vi "Enable.vi"(0 "reference in":refnum<class "Battery.lvclass">, 2 "Enable":bool, 5 "Error In":errorcluster) -> (14 "reference out":refnum<class "Battery.lvclass">, 19 "Error Out":errorcluster)   [LabVIEW 2023, in "Battery.lvclass"]
uses:
  Battery.lvclass
  Battery.lvclass/Battery.ctl
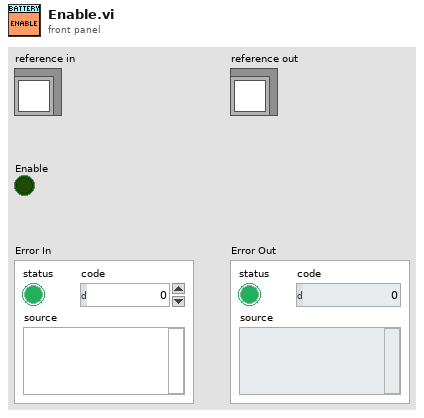
[diagram p1: front panel]
types:
  T1 = typedef "Battery.lvclass/ObjectAttributes.ctl" = cluster{"Python module":path, "Python Session":refnum<k35>, "PybammWrapper":refnum<k38>, "model loaded":bool, "simulation loaded":bool, "simulation enabled":bool, "SOC OCV Curve":dbl[][], "Open Circuit Voltage (V)":dbl, "State of Charge (%)":dbl, "HPS17K Refs":refnum<class "HPS-17000.lvclass">[], "# Cells in Series":u16, "# Cells in Parallel":u16, "Model Parameters":T2, "Simulation Parameters":T3}
  T2 = typedef "Battery.lvclass/Model Parameters.ctl" = cluster{"chemistry":string, "model_type":string}
  T3 = typedef "Battery.lvclass/Simulation Parameters.ctl" = cluster{"num_rc_pairs":i32, "R0":dbl, "R1":dbl, "C1":dbl, "R2":dbl, "C2":dbl, " nominal_capacity_Ah":dbl, "upper_voltage_cutoff":dbl, "lower_voltage_cutoff":dbl}
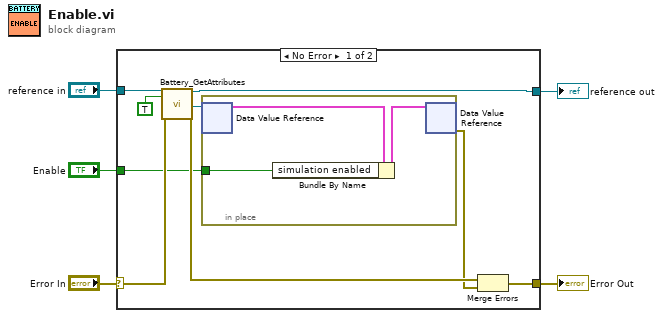
[diagram p0: block diagram]
diagram:
  n1 = case shown="No Error" "Error In" {
    selector: "Error In" -> [w14 w19]
    tunnel: [w12 w19] -> w4
    tunnel: [w6 w18] -> w2
    tunnel: "reference in" -> [w11 w18]
    tunnel: "Enable" -> [w8 _]
    frame No Error {
      n2 = call "Battery_GetAttributes.vi"("reference in"=w11, "OnlyGetDvrReference(False)"=TRUE, "Error In"=w14) -> ("reference out"=w6:refnum<class "Battery.lvclass">, "DataRef"=w9:refnum<data-value>, "Error Out"=w13:errorcluster)  [unwired: 13 in, 1 out]
      n3 = in-place {
        in-place-border: w8 -> [w17]
        n4 = in-place-dvr #1(w9) -> (w16:T1)  [unwired: 1 out]
        n5 = Bundle By Name(cluster=w16, "simulation enabled"=w17) -> (w15:T1)
        n6 = in-place-dvr #1(w15) -> (w7:errorcluster)  [unwired: 1 out]
      }
      n7 = Merge Errors(w13, w7) -> (w12:errorcluster)
    }
    frame Error {
    }
  }
  "Error Out" <- w4
  "reference out" <- w2
